vi "RT Main [RT].vi"   [LabVIEW 2017]
doc: "This template is for the Queued Message Handler design pattern.\n\nThe Event Handling Loop generates messages based on user interface actions.\n\nThe Message Handling Loop processes messages generated by the Event Handling Loop, or by other messages. The messages are string values, so new messages can be added easily to the Message Cases case structure in the Message Handling Loop. Each message cluster can also provide an optional value for Message Data, which is a variant that can be converted to whatever message-specific data is required."
uses:
  SubVIs/controls/Functional Global Operation.ctl
  SubVIs/controls/Control State.ctl
  SubVIs/controls/Raw Values.ctl
  SubVIs/controls/Control Configuration.ctl
  SubVIs/Globals/Global - RT Stream Connections.vi
  SubVIs/Globals/Global - Configuration Options.vi
  SubVIs/support/Message Queue/Message Queue.lvlib
  <vilib>/nisyscfg/nisyscfg.lvlib
panel:
  # "1) Ensure AI0..3 is wired to AO0...3 on TB1 and TB2.\n1) Run this VI first and ensure that it's running correctly.\n2) Run UI Main next.\n3) Input the IP address of the controller into UI Main's controller address control.\n4) Press connect on the UI Main's front panel."
types:
  T1 = typedef "Functional Global Operation.ctl" = enum16{"Initialize", "Read", "Write"}
  T2 = typedef "Control State.ctl" = enum16{"Safe State", "Control (PID)"}
  T3 = typedef "Raw Values.ctl" = cluster{"Channel 0":dbl, "Channel 1":dbl, "Channel 2":dbl, "Channel 3":dbl}
  T4 = typedef "Control Configuration.ctl" = cluster{"PID Gains":cluster{"proportional gain (Kc)":dbl, "integral gain (Kc*Ts/Ti)":dbl, "derivative gain (Kc*Td/Ts)":dbl}, "Output Range":cluster{"output high":dbl, "output low":dbl}}
  T5 = typedef "All Control Configuration Values.ctl" = cluster{"Control State":T2, "Setpoints":T3, "Control Configurations":T4[], "Temperature Thresholds":dbl[]}
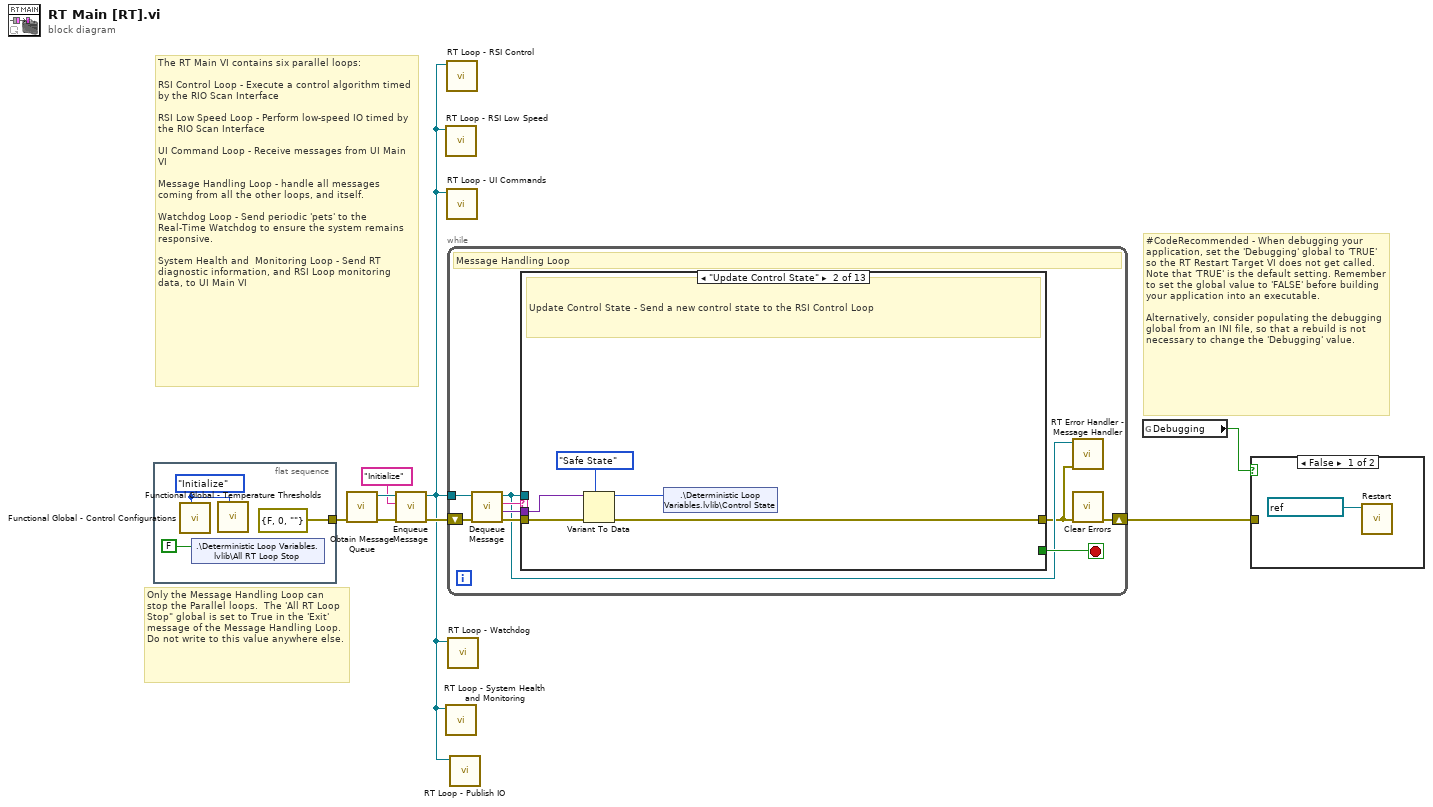
[diagram p0: block diagram]
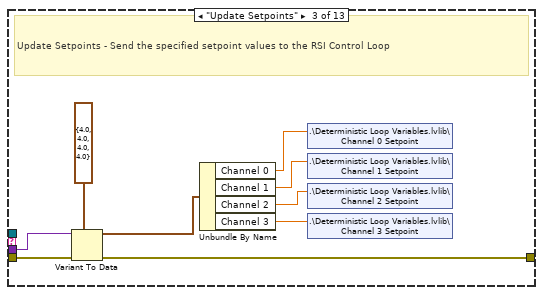
[diagram p4: hidden frame]
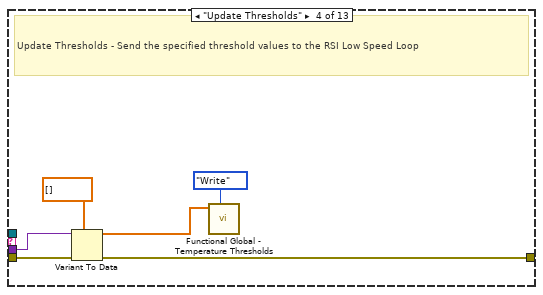
[diagram p5: hidden frame]
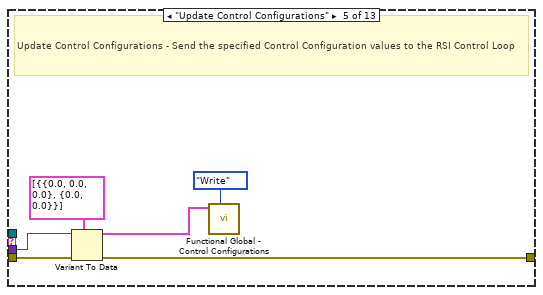
[diagram p6: hidden frame]
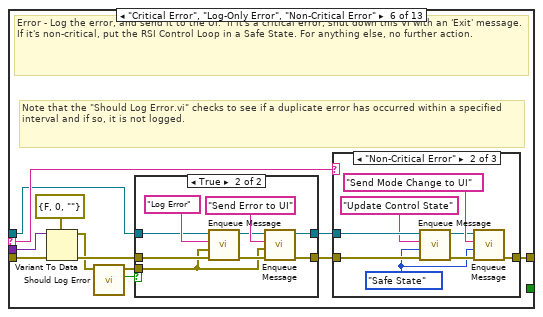
[diagram p7: hidden frame]
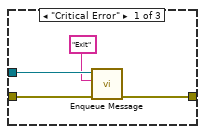
[diagram p9: hidden frame]
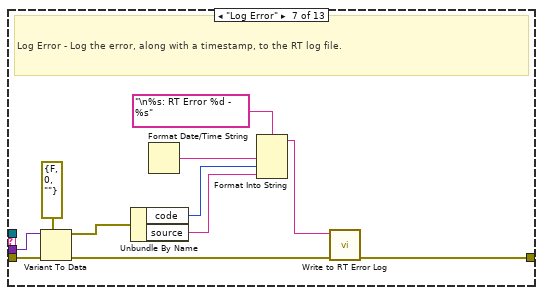
[diagram p11: hidden frame]
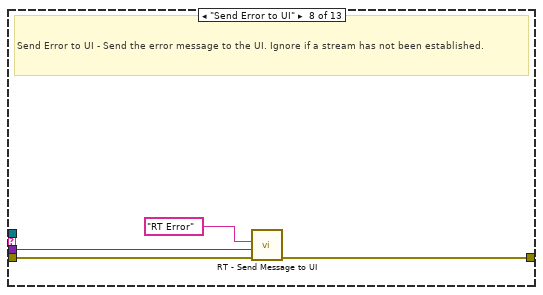
[diagram p12: hidden frame]
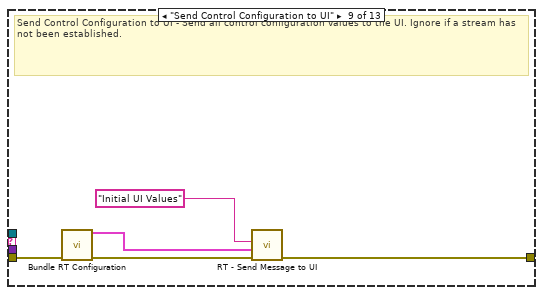
[diagram p13: hidden frame]
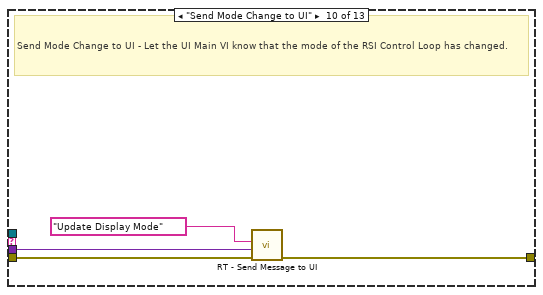
[diagram p14: hidden frame]
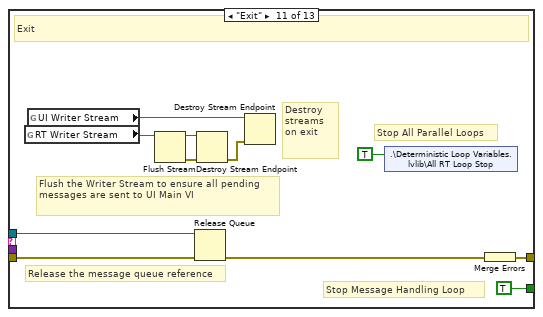
[diagram p15: hidden frame]
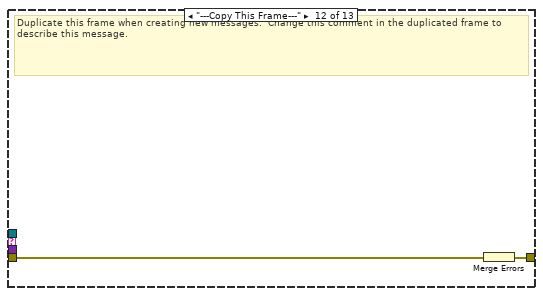
[diagram p16: hidden frame]
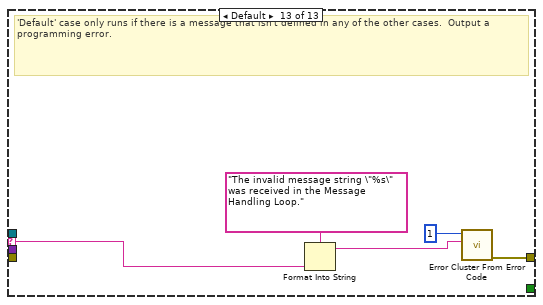
[diagram p17: hidden frame]
diagram:
  # "#CodeRecommended - When debugging your application, set the 'Debugging' global to 'TRUE' so the RT Restart Target VI does not get called.  Note that 'TRUE' is the default setting. Remember to set the global value to 'FALSE' before building your application into an executable.\n\nAlternatively, consider populating the debugging global from an INI file, so that a rebuild is not necessary to change the 'Debugging' value."
  # "The RT Main VI contains six parallel loops:\n\nRSI Control Loop - Execute a control algorithm timed by the RIO Scan Interface\n\nRSI Low Speed Loop - Perform low-speed IO timed by the RIO Scan Interface\n\nUI Command Loop - Receive messages from UI Main VI\n\nMessage Handling Loop - handle all messages coming from all the other loops, and itself.\n\nWatchdog Loop - Send periodic 'pets' to the Real-Time Watchdog to ensure the system remains responsive.\n\nSystem Health and  Monitoring Loop - Send RT diagnostic information, and RSI Loop monitoring data, to UI Main VI"
  # "Only the Message Handling Loop can stop the Parallel loops.  The 'All RT Loop Stop\" global is set to True in the 'Exit' message of the Message Handling Loop.  Do not write to this value anywhere else."
  n1 = flat-sequence {
    tunnel: [errorcluster {"status"=FALSE, "code"=0, "source"=""} ("error constant")] -> w4
    frame #0 {
      w10 = Functional_Global_Operation."Initialize" ("Functional Global Operation (Read)")
      n2 = call "Functional Global - Control Configurations.vi"("Functional Global Operation (Read)"=w10) -> ()  [unwired: 10 in, 1 out]
      n3 = shared-variable ".\\Deterministic Loop Variables.lvlib\\All RT Loop Stop"(FALSE) -> ()  [unwired: 1 in, 1 out]
      n4 = call "Functional Global - Temperature Thresholds.vi"("Functional Global Operation (Read)"=w10) -> ()  [unwired: 10 in, 1 out]
    }
  }
  n5 = call "Obtain Message Queue.vi"("error in (no error)"=w4) -> ("error out"=w2:errorcluster, "Message Queue"=w8:refnum<queue>)  [unwired: 9 in]
  n6 = call "Enqueue Message.vi"("error in (no error)"=w2, "Message"="Initialize", "Message Queue"=w8) -> ("error out"=w6:errorcluster, "dup Message Queue"=w1:refnum<queue>)  [unwired: 7 in]
  n7 = call "RT Loop - RSI Low Speed.vi"("Message Queue"=w1) -> ()  [unwired: 11 in]
  n8 = call "RT Loop - System Health and Monitoring.vi"("Message Queue"=w1) -> ()  [unwired: 11 in]
  n9 = call "RT Loop - RSI Control.vi"("Message Queue"=w1) -> ()  [unwired: 11 in]
  n10 = call "RT Loop - UI Commands.vi"("Message Queue"=w1) -> ()  [unwired: 11 in]
  n11 = while {
    tunnel: w1 -> [w15]
    shift-right: [w13] -> w3
    shift-left: w6 -> [w19]
    stop <- w20 stop-if-true
    # "Message Handling Loop"
    n12 = call "Dequeue Message.vi"("error in (no error)"=w19, "Message Queue"=w15) -> ("error out"=w18:errorcluster, "Message Data"=w16:variant, "Message"=w17:string, "dup Message Queue"=w14:refnum<queue>)  [unwired: 6 in]
    n13 = case "Message Cases" shown="\"Update Control State\"" w17 {
      selector: w17 -> [_ _ _ _ _ w57 _ _ _ _ _ _ w124]
      tunnel: w14 -> [_ _ _ _ _ w52 _ _ _ _ w118 _ _]
      tunnel: w18 -> [w21 w26 w35 w41 w47 w49 w94 w98 w103 w107 w114 w120 _]
      tunnel: [w21 w23 w27 w39 w44 w56 w85 w95 w99 w106 w115 w119 w122] -> w12
      tunnel: [_ _ _ _ _ _ _ _ _ _ TRUE _ _] -> w20
      tunnel: w16 -> [_ w25 w34 w40 w46 w55 w93 w97 _ w105 _ _ _]
      frame "Initialize" {
        # "Initialize - Currently a no-op for the RT Main VI"
      }
      frame "Update Control State" {
        # "Update Control State - Send a new control state to the RSI Control Loop"
        n14 = Variant To Data(error in=w26, type=Control_State."Safe State" ("FPGA State"), Variant=w25) -> (data=w22:T2, error out=w23:errorcluster)
        n15 = shared-variable ".\\Deterministic Loop Variables.lvlib\\Control State"(w22) -> ()  [unwired: 1 in, 1 out]
      }
      frame "Update Setpoints" {
        # "Update Setpoints - Send the specified setpoint values to the RSI Control Loop"
        n16 = Variant To Data(error in=w35, type=T3 {"Channel 0"=4.0, "Channel 1"=4.0, "Channel 2"=4.0, "Channel 3"=4.0} ("Raw Values"), Variant=w34) -> (data=w32:T3, error out=w27:errorcluster)
        n17 = Unbundle By Name(w32) -> ("Channel 0"=w28:dbl, "Channel 1"=w29:dbl, "Channel 2"=w30:dbl, "Channel 3"=w31:dbl)
        n18 = shared-variable ".\\Deterministic Loop Variables.lvlib\\Channel 0 Setpoint"(w28) -> ()  [unwired: 1 in, 1 out]
        n19 = shared-variable ".\\Deterministic Loop Variables.lvlib\\Channel 1 Setpoint"(w29) -> ()  [unwired: 1 in, 1 out]
        n20 = shared-variable ".\\Deterministic Loop Variables.lvlib\\Channel 2 Setpoint"(w30) -> ()  [unwired: 1 in, 1 out]
        n21 = shared-variable ".\\Deterministic Loop Variables.lvlib\\Channel 3 Setpoint"(w31) -> ()  [unwired: 1 in, 1 out]
      }
      frame "Update Thresholds" {
        # "Update Thresholds - Send the specified threshold values to the RSI Low Speed Loop"
        n22 = Variant To Data(error in=w41, type=dbl[] [], Variant=w40) -> (data=w36:dbl[], error out=w39:errorcluster)
        n23 = call "Functional Global - Temperature Thresholds.vi"("Functional Global Operation (Read)"=Functional_Global_Operation."Write", "Temperature Thresholds in"=w36) -> ()  [unwired: 9 in, 1 out]
      }
      frame "Update Control Configurations" {
        # "Update Control Configurations - Send the specified Control Configuration values to the RSI Control Loop"
        n24 = Variant To Data(error in=w47, type=T4[] [{"PID Gains"={"proportional gain (Kc)"=0.0, "integral gain (Kc*Ts/Ti)"=0.0, "derivative gain (Kc*Td/Ts)"=0.0}, "Output Range"={"output high"=0.0, "output low"=0.0}}], Variant=w46) -> (data=w43:T4[], error out=w44:errorcluster)
        n25 = call "Functional Global - Control Configurations.vi"("Functional Global Operation (Read)"=Functional_Global_Operation."Write", "Control Configurations in"=w43) -> ()  [unwired: 9 in, 1 out]
      }
      frame "Critical Error", "Log-Only Error", "Non-Critical Error" {
        # "Note that the \"Should Log Error.vi\" checks to see if a duplicate error has occurred within a specified interval and if so, it is not logged."
        # "Error - Log the error, and send it to the UI.  If it's a critical error, shut down this VI with an 'Exit' message. If it's non-critical, put the RSI Control Loop in a Safe State. For anything else, no further action."
        n26 = Variant To Data(error in=w49, type=errorcluster {"status"=FALSE, "code"=0, "source"=""} ("error out"), Variant=w55) -> (data=w48:errorcluster, error out=w53:errorcluster)
        n27 = call "Should Log Error.vi"("error to report"=w48) -> ("Should Log Error?"=w51:bool, "dup error to report"=w50:errorcluster)  [unwired: 9 in]
        n28 = case shown="True" w51 {
          tunnel: [w61 w68] -> w59
          tunnel: [w60 w67] -> w58
          tunnel: w52 -> [w60 w66]
          tunnel: w53 -> [w61 w63]
          tunnel: w50 -> [_ w62]
          frame False {
          }
          frame True {
            n29 = call "Enqueue Message.vi"("error in (no error)"=w63, "Message Data"=w62, "Message"="Log Error", "Message Queue"=w66) -> ("error out"=w64:errorcluster, "dup Message Queue"=w65:refnum<queue>)  [unwired: 6 in]
            n30 = call "Enqueue Message.vi"("error in (no error)"=w64, "Message Data"=w62, "Message"="Send Error to UI", "Message Queue"=w65) -> ("error out"=w68:errorcluster, "dup Message Queue"=w67:refnum<queue>)  [unwired: 6 in]
          }
        }
        n31 = case shown="\"Non-Critical Error\"" w57 {
          tunnel: w59 -> [w74 w82 w83]
          tunnel: w58 -> [w72 w81 _]
          tunnel: [w73 w78 w83] -> w56
          frame "Critical Error" {
            n32 = call "Enqueue Message.vi"("error in (no error)"=w74, "Message"="Exit", "Message Queue"=w72) -> ("error out"=w73:errorcluster)  [unwired: 7 in, 1 out]
          }
          frame "Non-Critical Error" {
            w75 = Control_State."Safe State" ("FPGA State")
            n33 = call "Enqueue Message.vi"("error in (no error)"=w82, "Message Data"=w75, "Message"="Update Control State", "Message Queue"=w81) -> ("error out"=w79:errorcluster, "dup Message Queue"=w76:refnum<queue>)  [unwired: 6 in]
            n34 = call "Enqueue Message.vi"("error in (no error)"=w79, "Message Data"=w75, "Message"="Send Mode Change to UI", "Message Queue"=w76) -> ("error out"=w78:errorcluster)  [unwired: 6 in, 1 out]
          }
          frame Default {
          }
        }
      }
      frame "Log Error" {
        # "Log Error - Log the error, along with a timestamp, to the RT log file."
        n35 = Variant To Data(error in=w94, type=errorcluster {"status"=FALSE, "code"=0, "source"=""} ("error constant"), Variant=w93) -> (data=w88:errorcluster, error out=w91:errorcluster)
        n36 = Unbundle By Name(w88) -> ("code"=w87:i32, "source"=w86:string)
        n37 = Format Date/Time String() -> (date/time string=w89:string)  [unwired: 3 in]
        n38 = Format Into String(format string="\n%s: RT Error %d - %s", w89, w87, w86) -> (resulting string=w84:string)  [unwired: 2 in, 1 out]
        n39 = call "Write to RT Error Log.vi"("error in (no error)"=w91, "Log Entry"=w84) -> ("error out"=w85:errorcluster)  [unwired: 9 in]
      }
      frame "Send Error to UI" {
        # "Send Error to UI - Send the error message to the UI. Ignore if a stream has not been established."
        n40 = call "RT - Send Message to UI.vi"("error in (no error)"=w98, "Message Data"=w97, "Message"="RT Error") -> ("error out"=w95:errorcluster)  [unwired: 8 in]
      }
      frame "Send Control Configuration to UI" {
        # "Send Control Configuration to UI - Send all control configuration values to the UI. Ignore if a stream has not been established."
        n41 = call "Bundle RT Configuration.vi"("error in (no error)"=w103) -> ("error out"=w102:errorcluster, "All Control Configuration Values"=w101:T5)  [unwired: 9 in]
        n42 = call "RT - Send Message to UI.vi"("error in (no error)"=w102, "Message Data"=w101, "Message"="Initial UI Values") -> ("error out"=w99:errorcluster)  [unwired: 8 in]
      }
      frame "Send Mode Change to UI" {
        # "Send Mode Change to UI - Let the UI Main VI know that the mode of the RSI Control Loop has changed."
        n43 = call "RT - Send Message to UI.vi"("error in (no error)"=w107, "Message Data"=w105, "Message"="Update Display Mode") -> ("error out"=w106:errorcluster)  [unwired: 8 in]
      }
      frame "Exit" {
        # "Flush the Writer Stream to ensure all pending messages are sent to UI Main VI"
        # "Destroy streams on exit"
        # "Stop Message Handling Loop"
        # "Stop All Parallel Loops"
        # "Release the message queue reference"
        # "Exit"
        n44 = global read "Global - RT Stream Connections.vi" "RT Writer Stream"() -> (w113:refnum<k21>)
        n45 = global read "Global - RT Stream Connections.vi" "UI Writer Stream"() -> (w112:refnum<k21>)
        n46 = Flush Stream(11:w113) -> (0:w108:errorcluster, 3:w109:refnum<k21>)  [unwired: 3 in, 1 out]
        n47 = Release Queue(queue=w118, error in (no error)=w114) -> (error out=w116:errorcluster)  [unwired: 1 in, 2 out]
        n48 = Destroy Stream Endpoint(8:w108, 11:w109) -> (0:w111:errorcluster)
        n49 = Destroy Stream Endpoint(8:w111, 11:w112) -> ()  [unwired: 1 out]
        n50 = shared-variable ".\\Deterministic Loop Variables.lvlib\\All RT Loop Stop"(TRUE ("Stop Monitoring Loops")) -> ()  [unwired: 1 in, 1 out]
        n51 = Merge Errors(w116) -> (w115:errorcluster)
      }
      frame "---Copy This Frame---" {
        # "Duplicate this frame when creating new messages.  Change this comment in the duplicated frame to describe this message."
        n52 = Merge Errors(w120) -> (w119:errorcluster)
      }
      frame Default {
        # "'Default' case only runs if there is a message that isn't defined in any of the other cases.  Output a programming error."
        n53 = Format Into String(format string="The invalid message string \"%s\" was received in the Message Handling Loop." ("Unknown Message Error Text"), w124) -> (resulting string=w121:string)  [unwired: 2 in, 1 out]
        n54 = call <vilib>:"Error Cluster From Error Code.vi"("error message (\"\")"=w121, "error code (0)"=1) -> ("error out"=w122:errorcluster)  [unwired: 7 in]
      }
    }
    n55 = call "RT Error Handler - Message Handler.vi"("error in (no error)"=w12, "Message Queue"=w14) -> ()  [unwired: 9 in, 1 out]
    n56 = call <vilib>:"Clear Errors.vi"("error in (no error)"=w12) -> ("error out"=w13:errorcluster)  [unwired: 5 in, 1 out]
  }
  n57 = call "RT Loop - Watchdog.vi"("Message Queue"=w1) -> ()  [unwired: 11 in]
  n58 = call "RT Loop - Publish IO.vi"("Message Queue"=w1) -> ()  [unwired: 11 in]
  n59 = global read "Global - Configuration Options.vi" "Debugging"() -> (w5:bool)
  n60 = case shown="False" w5 {
    tunnel: w3 -> [_ _]
    frame False {
      n61 = call <vilib>:"Restart.vi"("Session in"=refnum<k21> "localhost" ("session in")) -> ()  [unwired: 8 in, 3 out]
    }
    frame True {
    }
  }
